vi "Get VIRef from ClassItem.vi"(8 "error in (no error)":errorcluster, 10 "item name":string, 11 "class in":refnum<vi>) -> (0 "error out":errorcluster, 1 "found":bool, 2 "vi":refnum<vi>, 3 "class out":refnum<vi>)   [LabVIEW 2019, in "gRPC Template Creation Utility.lvlib"]
uses:
  gRPC Template Creation Utility.lvlib
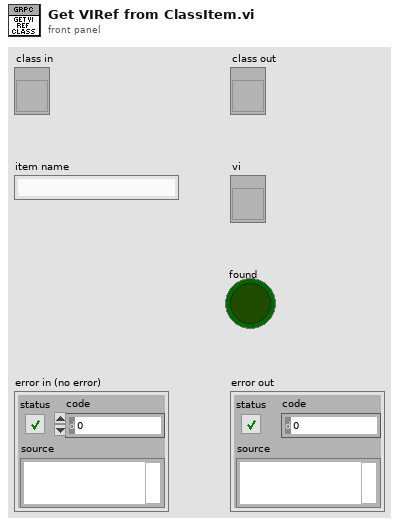
[diagram p1: front panel]
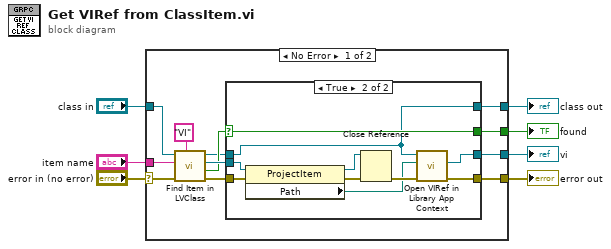
[diagram p0: block diagram]
diagram:
  n1 = case shown="No Error" "error in (no error)" {
    selector: "error in (no error)" -> [w13 w33]
    tunnel: "class in" -> [w17 w34]
    tunnel: "item name" -> [w15 _]
    tunnel: [w9 w34] -> w2
    tunnel: [w14 w33] -> w4
    tunnel: [w11 _] -> w3
    tunnel: [w8 _] -> w1
    frame No Error {
      n2 = call "Find Item in LVClass.vi"("Item Type"="VI", "error in (no error)"=w13, "Item Name"=w15, "Class Item in"=w17) -> ("error out"=w19:errorcluster, "Found?"=w12:bool, "Project Item (Class Item)"=w18:refnum<vi>, "Class Item out"=w10:refnum<vi>)  [unwired: 4 in]
      n3 = case shown="True" w12 {
        selector: w12 -> [w21 w30]
        tunnel: w19 -> [w22 w32]
        tunnel: w18 -> [_ w31]
        tunnel: [w22 w25] -> w14
        tunnel: [w21 w30] -> w11
        tunnel: w10 -> [w20 w23]
        tunnel: [w20 w23] -> w9
        tunnel: [_ w24] -> w8
        frame False {
        }
        frame True {
          n4 = property class="ProjectItem"(reference=w31, error in=w32) -> (reference out=w28:refnum<vi>, error out=w29:errorcluster, "Path"=w26:path)
          n5 = Close Reference(reference=w28, error in (no error)=w29) -> (error out=w27:errorcluster)
          n6 = call "Open VIRef in Library App Context.vi"("error in (no error)"=w27, "vi path"=w26, "library in"=w23) -> ("error out"=w25:errorcluster, "vi"=w24:refnum<vi>)  [unwired: 6 in, 1 out]
        }
      }
    }
    frame Error {
    }
  }
  "class out" <- w2
  "error out" <- w4
  "found" <- w3
  "vi" <- w1
